vi "myXi_InitializeStartBust.vi"(5 "subwindow IN":refnum<vi>, 7 "queue size":i32, 8 "error in (no error)":errorcluster, 10 "image frames":i64=100, 11 "xiCam IN":refnum<k24>) -> (0 "error out":errorcluster, 2 "Array":u8[](array[numeric]), 3 "xiCam Out":refnum<k24>)   [LabVIEW 2018]
uses:
  C:/XIMEA/API/x64/xiApi.NETX64.dll
  VisionLibrariesXimea/xiLib/xiLIB_64bit/xiLIB/xiCamLib/xiCam/PRM/PRM/PRM_v2.ctl
  VisionLibrariesXimea/xiLib/xiLIB_64bit/xiLIB/xiCamLib/xiCam/PRM/TRG_SOURCE/TRG_SOURCE.ctl
  VisionLibrariesXimea/xiLib/xiLIB_64bit/xiLIB/xiCamLib/xiCam/PRM/TRG_SELECTOR/TRG_SELECTOR.ctl
  VisionLibrariesXimea/xiLib/xiLIB_64bit/xiLIB/xiCamLib/xiLIB/xiLIB - GetPRM_INFO.vi
  VisionLibrariesXimea/xiLib/xiLIB_64bit/xiLIB/xiCamLib/xiCam/Methods/xiCam - GetParam_Float.vi
  VisionLibrariesXimea/xiLib/xiLIB_64bit/xiLIB/xiCamLib/xiCam/Methods/xiCam - GetParam_String.vi
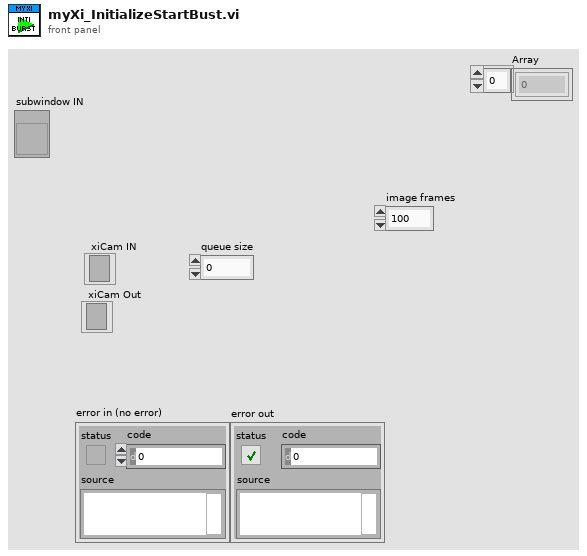
[diagram p1: front panel]
types:
  T1 = typedef "LVPointDoubleTypeDef.ctl" = cluster{"X":dbl, "Y":dbl}
  T2 = cluster{"2^n : x":i8, "2^n : y":i8, "lower left box Position":T1, "Height":i32, "Width":i32}
  T3 = typedef "PRM_v2.ctl" = enum16{"ACQ_BUFFER_SIZE", "ACQ_FRAME_BURST_COUNT", "ACQ_TIMING_MODE", "ACQ_TRANSPORT_BUFFER_SIZE", "AE_MAX_LIMIT", "AEAG", "AEAG_LEVEL", "API_VERSION", "AG_MAX_LIMIT", "APPLY_CMS", "AUTO_BANDWIDTH_CALCULATION", "AUTO_WB", "AVAILABLE_BANDWIDTH", "AVAILABLE_BANDWIDTH_MAX", "AVAILABLE_BANDWIDTH_MIN", "BPC", "BUFFER_POLICY", "BUFFERS_QUEUE_SIZE", "CC_MATRIX_00", "CC_MATRIX_01", "CC_MATRIX_02", "CC_MATRIX_03", "CC_MATRIX_10", "CC_MATRIX_11", "CC_MATRIX_12", "CC_MATRIX_13", "CC_MATRIX_20", "CC_MATRIX_21", "CC_MATRIX_22", "CC_MATRIX_23", "CC_MATRIX_30", "CC_MATRIX_31", "CC_MATRIX_32", "CC_MATRIX_33", "CHIP_TEMP", "CMS", "COLOR_FILTER_ARRAY", "COOLING", "DEBOUNCE_EN", "DEBOUNCE_POL", "DEBOUNCE_T0", "DEBOUNCE_T1", "DEBUG_LEVEL", "DEFAULT_CC_MATRIX", "DEVICE_INSTANCE_PATH", "DEVICE_MODEL_ID", "DEVICE_NAME", "DEVICE_SN", "DEVICE_TYPE", "DEVICE_USER_ID", "DOWNSAMPLING", "DOWNSAMPLING_MAX", "DOWNSAMPLING_MIN", "DOWNSAMPLING_TYPE", "DRV_VERSION", "EXP_PRIORITY", "EXPOSURE", "EXPOSURE_DIRECT_UPDATE", "EXPOSURE_MAX", "EXPOSURE_MIN", "FFS_FILE_NAME", "FPGA1_VERSION", "FRAMERATE", "FRAMERATE_MAX", "FRAMERATE_MIN", "FREE_FFS_SIZE", "GAIN", "GAIN_DIRECT_UPDATE", "GAIN_MAX", "GAIN_MIN", "GAMMAC", "GAMMAY", "GPI_LEVEL", "GPI_MODE", "GPI_SELECTOR", "GPI_SELECTOR_MAX", "GPI_SELECTOR_MIN", "GPO_MODE", "GPO_SELECTOR", "GPO_SELECTOR_MAX", "GPO_SELECTOR_MIN", "HDR", "HDR_T1", "HDR_T2", "HEIGHT", "HEIGHT_MAX", "HEIGHT_MIN", "HOUSE_TEMP", "IMAGE_DATA_FORMAT", "IMAGE_IS_COLOR", "INPUT_CMS_PROFILE", "IS_COOLED", "IS_DEVICE_EXIST", "KNEEPOINT1", "KNEEPOINT2", "LED_MODE", "LED_SELECTOR", "LED_SELECTOR_MAX", "LED_SELECTOR_MIN", "LIMIT_BANDWIDTH", "LIMIT_BANDWIDTH_MAX", "LIMIT_BANDWIDTH_MIN", "LUT_EN", "LUT_INDEX", "LUT_INDEX_MAX", "LUT_INDEX_MIN", "LUT_VALUE", "LUT_VALUE_MAX", "LUT_VALUE_MIN", "MANUAL_WB", "MCU1_VERSION", "MCU2_VERSION", "OFFSET_X", "OFFSET_X_MAX", "OFFSET_X_MIN", "OFFSET_Y", "OFFSET_Y_MAX", "OFFSET_Y_MIN", "OUTPUT_CMS_PROFILE", "OUTPUT_DATA_BIT_DEPTH", "OUTPUT_DATA_PACKING", "READ_FILE_FFS", "RECENT_FRAME", "SENSOR_DATA_BIT_DEPTH", "SENSOR_MODE", "SENSOR_TAPS", "SHARPNESS", "SHUTTER_TYPE", "TARGET_TEMP", "TRG_DELAY", "TRG_SELECTOR", "TRG_SOFTWARE", "TRG_SOURCE", "USED_FFS_SIZE", "WB_KB", "WB_KG", "WB_KR", "WIDTH", "WIDTH_MAX", "WIDTH_MIN", "WRITE_FILE_FFS", "ACQ_BUFFER_SIZE_UNIT", "ACQ_TRANSPORT_BUFFER_COMMIT", "AEAG_ROI_HEIGHT", "AEAG_ROI_OFFSET_X", "AEAG_ROU_OFFSET_Y", "AEAG_ROI_WIDTH", "API_CONTEXT_LIST", "BINNING_HORIZONTAL", "BINNING_SELECTOR", "BINNING_VERTICAL", "COLUMN_FPN_CORRECTION", "COUNTER_SELECTOR", "COUNTER_VALUE", "DECIMATION_HORIZONTAL", "DECIMATION_SELECTOR", "DECIMATION_VERTICAL", "DEVICE_ID", "DEVICE_LOCATION_PATH", "DEVICE_MANIFEST", "DEVICE_RESET", "DEVICE_SENS_SN", "EXPOSURE_BURST_COUNT", "FFS_ACCESS_KEY", "GAIN_SELECTOR", "HW_REVISION", "IMAGE_BLACK_LEVEL", "IMAGE_DATA_BIT_DEPTH", "IMAGE_DATA_FORMAT_RGB32_ALPHA", "IMAGE_PAYLOAD_SIZE", "LENS_APERTURE_VALUE", "LENS_FEATURE", "LENS_FEATURE_SELECTOR", "LENS_FOCAL_LENGTH", "LENS_FOCUS_DISTANCE", "LENS_FOCUS_MOVE", "LENS_FOCUS_MOVEMENT_VALUE", "LENS_MODE", "OUTPUT_DATA_PACKING_TYPE", "SENSOR_CLOCK_FREQ_HZ", "SENSOR_CLOCK_FREQ_INDEX", "SENSOR_FEATURE_SELECTOR", "SENSOR_FEATURE_VALUE", "SENSOR_OUTPUT_CHANNEL_COUNT", "TRANSPORT_PIXEL_FORMAT", "TS_RST_MODE", "TS_RST_SOURCE"}
  T4 = typedef "TRG_SOURCE.ctl" = enum16{"OFF", "EDGE_RISING", "EDGE_FALLING", "SOFTWARE"}
  T5 = typedef "TRG_SELECTOR.ctl" = enum16{"FRAME_START", "EXPOSURE_ACTIVE", "FRAME_BURST_START", "FRAME_BURST_ACTIVE"}
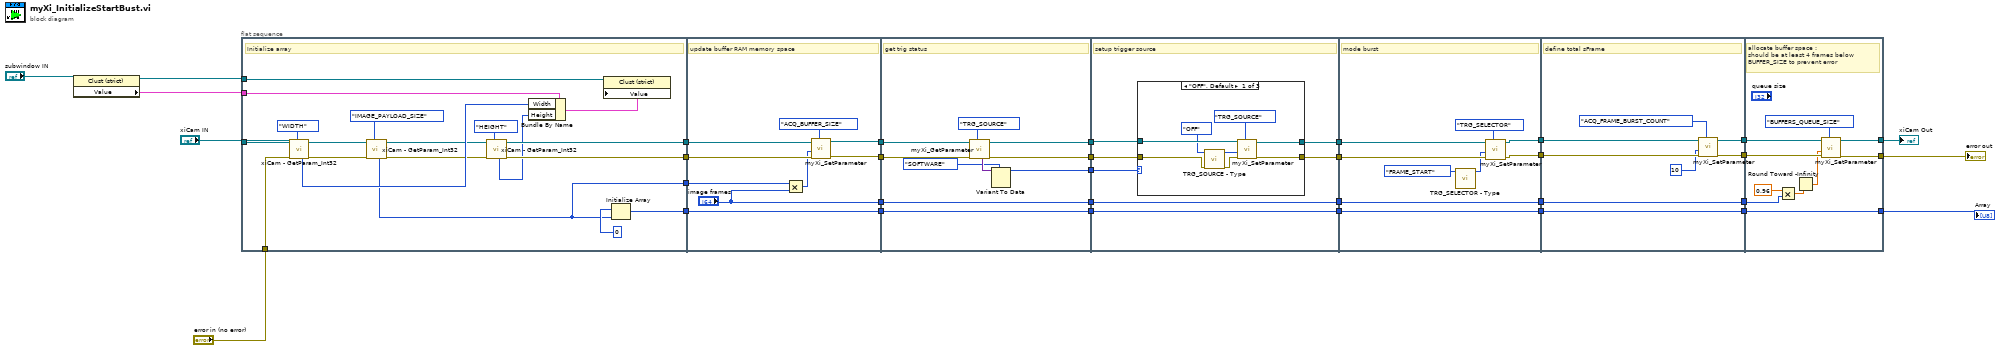
[diagram p0: block diagram]
diagram:
  n1 = property class="Clust (strict)"(reference="subwindow IN") -> (reference out=w7:refnum<vi>, "Value"=w8:T2)  [unwired: 1 in, 1 out]
  n2 = flat-sequence {
    tunnel: "xiCam IN" -> [w52]
    tunnel: [w49] -> w19
    tunnel: "error in (no error)" -> [w48]
    tunnel: [w47] -> w18
    tunnel: [w45] -> w17
    tunnel: w8 -> [w42]
    tunnel: w7 -> [w40]
    tunnel: [w34] -> w6
    tunnel: w19 -> [w59]
    tunnel: [w58] -> w16
    tunnel: w18 -> [w61]
    tunnel: [w60] -> w14
    tunnel: w17 -> [w56]
    tunnel: [w56] -> w12
    tunnel: w6 -> [w54]
    tunnel: ["image frames"] -> w5
    tunnel: w16 -> [w68]
    tunnel: [w67] -> w15
    tunnel: w14 -> [w70]
    tunnel: [w69] -> w13
    tunnel: w12 -> [w71]
    tunnel: [w71] -> w11
    tunnel: [w63] -> w10
    tunnel: w5 -> [w62]
    tunnel: [w62] -> w4
    tunnel: [w77] -> w32
    tunnel: [w76] -> w31
    tunnel: w15 -> [w78]
    tunnel: w13 -> [w75]
    tunnel: [w74] -> w21
    tunnel: w11 -> [w74]
    tunnel: w10 -> [w73]
    tunnel: w4 -> [w72]
    tunnel: [w72] -> w3
    tunnel: w32 -> [w98]
    tunnel: w31 -> [w97]
    tunnel: [w94] -> w30
    tunnel: [w93] -> w29
    tunnel: [w92] -> w22
    tunnel: w21 -> [w92]
    tunnel: w3 -> [w91]
    tunnel: [w91] -> w2
    tunnel: w30 -> [w107]
    tunnel: w29 -> [w106]
    tunnel: [w104] -> w28
    tunnel: [w103] -> w27
    tunnel: [w102] -> w23
    tunnel: w22 -> [w102]
    tunnel: w2 -> [w100]
    tunnel: [w100] -> w1
    tunnel: w28 -> [w117]
    tunnel: w27 -> [w115]
    tunnel: [w114] -> w25
    tunnel: [w113] -> w26
    tunnel: [w112] -> w20
    tunnel: w23 -> [w112]
    tunnel: w1 -> [w111]
    frame #0 {
      # "Initialize array"
      n3 = call "xiCam - GetParam_Int32.vi"("PRM"=PRM_v2."WIDTH", "error in (no error)"=w48, "xiCam In"=w52) -> ("error out"=w36:errorcluster, "xiCam Out"=w39:refnum<k24>, "Int32_Value"=w44:i32)  [unwired: 6 in]
      n4 = call "xiCam - GetParam_Int32.vi"("PRM"=PRM_v2."IMAGE_PAYLOAD_SIZE", "error in (no error)"=w36, "xiCam In"=w39) -> ("error out"=w35:errorcluster, "xiCam Out"=w38:refnum<k24>, "Int32_Value"=w34:i32)  [unwired: 6 in]
      n5 = call "xiCam - GetParam_Int32.vi"("PRM"=PRM_v2."HEIGHT", "error in (no error)"=w35, "xiCam In"=w38) -> ("error out"=w47:errorcluster, "xiCam Out"=w49:refnum<k24>, "Int32_Value"=w43:i32)  [unwired: 6 in]
      n6 = Bundle By Name(cluster=w42, "Width"=w44, "Height"=w43) -> (w41:T2)
      n7 = property class="Clust (strict)"(reference=w40, "Value"=w41) -> ()  [unwired: 1 in, 2 out]
      n8 = Initialize Array "Initialize Array"(u8 0 ("element"), w34) -> (w45:u8[])
    }
    frame #1 {
      # "update buffer RAM memory space"
      n9 = Multiply(x=w54, y="image frames") -> (x*y=w55:i64)
      n10 = call "myXi_SetParameter.vi"("input PRM"=PRM_v2."ACQ_BUFFER_SIZE", "error in"=w61, "input value I32"=w55, "xiCam IN"=w59) -> ("error out"=w60:errorcluster, "xiCam Out"=w58:refnum<k24>)  [unwired: 6 in]
    }
    frame #2 {
      # "get trig status"
      n11 = call "myXi_GetParameter.vi"("input PRM"=PRM_v2."TRG_SOURCE", "error in"=w70, "xiCam IN"=w68) -> ("error out"=w69:errorcluster, "xiCam Out"=w67:refnum<k24>, "output"=w65:variant)  [unwired: 3 in, 3 out]
      n12 = Variant To Data(type=TRG_SOURCE."SOFTWARE" ("TRG_SOURCE"), Variant=w65) -> (data=w63:T4)  [unwired: 1 in, 1 out]
    }
    frame #3 {
      # "setup trigger source"
      n13 = case shown="\"OFF\", Default" w73 {
        tunnel: w78 -> [w86 w88 w90]
        tunnel: [w85 w87 w89] -> w77
        tunnel: [w84 w88 w90] -> w76
        tunnel: w75 -> [w83 w87 w89]
        frame "OFF", Default {
          n14 = call "TRG_SOURCE - Type.vi"("error in (no error)"=w83, "TRG_SOURCE"=TRG_SOURCE."OFF") -> ("error out"=w80:errorcluster, "TRG_SOURCE_VALUE"=w81:i32)  [unwired: 8 in]
          n15 = call "myXi_SetParameter.vi"("input PRM"=PRM_v2."TRG_SOURCE", "error in"=w80, "input value I32"=w81, "xiCam IN"=w86) -> ("error out"=w85:errorcluster, "xiCam Out"=w84:refnum<k24>)  [unwired: 6 in]
        }
        frame "EDGE_RISING" {
        }
        frame "EDGE_FALLING" {
        }
      }
    }
    frame #4 {
      # "mode burst"
      n16 = call "TRG_SELECTOR - Type.vi"("TRG_SELECTOR"=TRG_SELECTOR."FRAME_START") -> ("TRG_SELECTOR_VALUE"=w95:i32)  [unwired: 9 in, 1 out]
      n17 = call "myXi_SetParameter.vi"("input PRM"=PRM_v2."TRG_SELECTOR", "error in"=w98, "input value I32"=w95, "xiCam IN"=w97) -> ("error out"=w93:errorcluster, "xiCam Out"=w94:refnum<k24>)  [unwired: 6 in]
    }
    frame #5 {
      # "define total sFrame"
      n18 = call "myXi_SetParameter.vi"("input PRM"=PRM_v2."ACQ_FRAME_BURST_COUNT", "error in"=w106, "input value I32"=10 ("burst count"), "xiCam IN"=w107) -> ("error out"=w103:errorcluster, "xiCam Out"=w104:refnum<k24>)  [unwired: 6 in]
    }
    frame #6 {
      # "allocate buffer space : \nshould be at least 4 frames below \nBUFFER_SIZE to prevent error"
      n19 = Multiply(x=0.96, y=w111) -> (x*y=w109:dbl)
      n20 = Round Toward -Infinity(1:w109) -> (0:w108:dbl)
      n21 = call "myXi_SetParameter.vi"("input PRM"=PRM_v2."BUFFERS_QUEUE_SIZE", "error in"=w115, "input value I32"=w108, "xiCam IN"=w117) -> ("error out"=w114:errorcluster, "xiCam Out"=w113:refnum<k24>)  [unwired: 6 in]
    }
  }
  "xiCam Out" <- w26
  "error out" <- w25
  "Array" <- w20
